vi "Betonauswahl.vi"(8 "error in (no error)":errorcluster) -> (0 "error out":errorcluster)   [LabVIEW 2023]
doc: "Diese Vi liest das Config file und errechnet den Preis pro menge für die Betonsorte \nErsstellt: Mustafa Khaki\nDatum: 12.11.2025"
uses:
  CONTROLS/Betonauswahl.ctl
  <vilib>/Utility/miscctls.llb/LVRectTypeDef.ctl
panel:
  out "Preis":dbl
  in  "Betonauswahl":T1
  in  "Menge":dbl
  in  "Blank Button 2":bool
  in  "Blank Button":bool
  in  "Reserve schalter":bool
  in  "Stop Button":bool
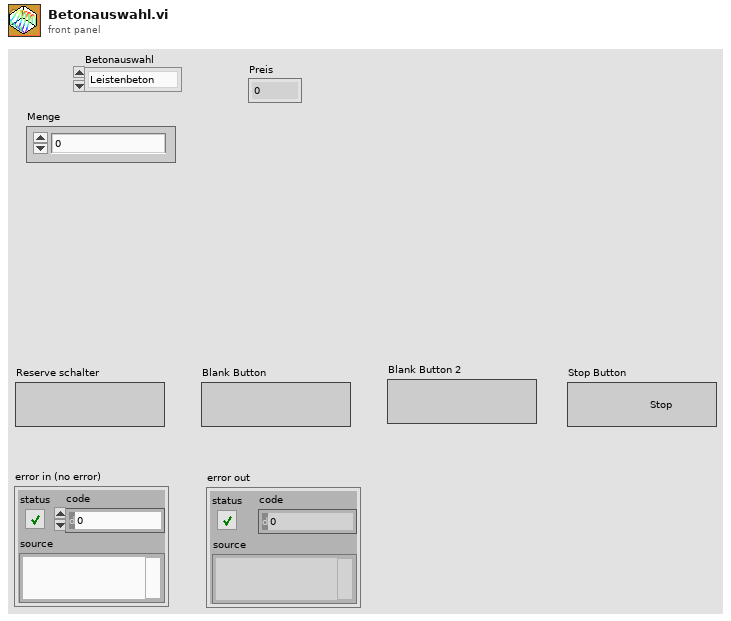
[diagram p1: front panel]
types:
  T1 = typedef "Betonauswahl.ctl" = enum16{"Leistenbeton", "Erdfeuchter Beton", "Beton", "Erdfeuchter Starker Beton", "Starker Beton"}
  T2 = typedef "LVRectTypeDef.ctl" = cluster{"Left":i16, "Top":i16, "Right":i16, "Bottom":i16}
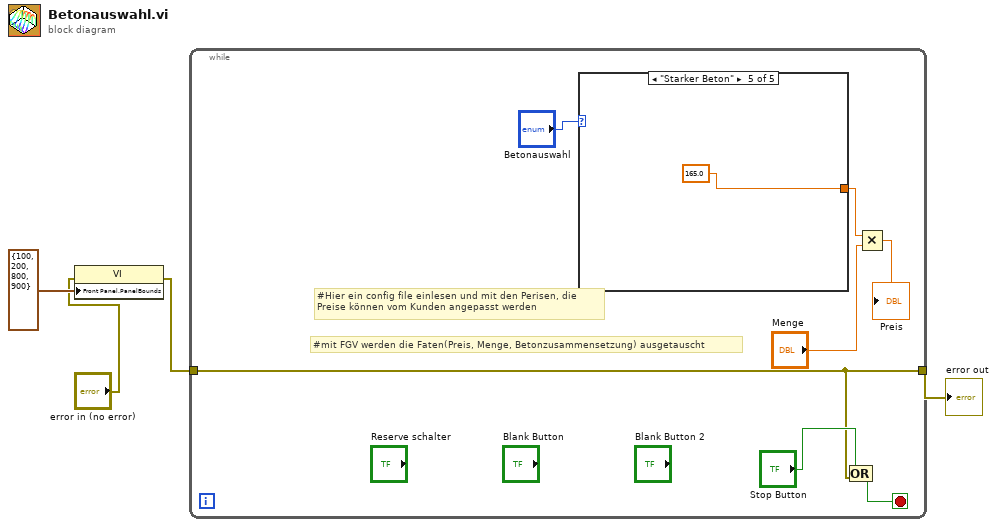
[diagram p0: block diagram]
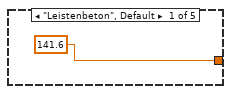
[diagram p2: hidden frame]
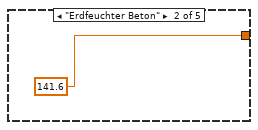
[diagram p3: hidden frame]
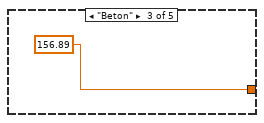
[diagram p4: hidden frame]
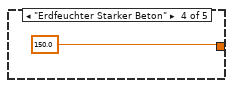
[diagram p5: hidden frame]
diagram:
  n1 = property class="VI"(error in="error in (no error)", "Front Panel.PanelBounds"=T2 {"Left"=100, "Top"=200, "Right"=800, "Bottom"=900} ("Front Panel Window:Panel Bounds")) -> (error out=w1:errorcluster)  [unwired: 1 in, 1 out]
  n2 = while {
    tunnel: [w9] -> w4
    tunnel: w1 -> [w9]
    stop <- w10 stop-if-true
    # "#mit FGV werden die Faten(Preis, Menge, Betonzusammensetzung) ausgetauscht"
    # "#Hier ein config file einlesen und mit den Perisen, die \nPreise können vom Kunden angepasst werden"
    n3 = case shown="\"Starker Beton\"" "Betonauswahl" {
      tunnel: [141.6 141.6 156.89 150.0 165.0] -> w7
      frame "Leistenbeton", Default {
      }
      frame "Erdfeuchter Beton" {
      }
      frame "Beton" {
      }
      frame "Erdfeuchter Starker Beton" {
      }
      frame "Starker Beton" {
      }
    }
    n4 = Compound Arithmetic op=OR("Stop Button", w9) -> (w10:bool)
    n5 = Multiply(x=w7, y="Menge") -> (x*y=→"Preis":dbl)
  }
  "error out" <- w4
